vi "BuildCustomDashBoardData.vi"() -> ()   [LabVIEW 2013]
doc: "This VI builds data and sends it back to the dashboard PC program. By default it sends back the raw values for the first analog, digital, and solenoid module. Modify it to send back the data you want to view. Consider adding higher level data to the Dashboard Datatype.ctl and to this VI. Then update the Dashboard to display the data however you like.\n\nThis software is licensed. Open the labview\\readme\\WPI Robotics Library Open Source License.txt file for more information."
uses:
  typedefs/dashboard/DashboardEnable.ctl
  typedefs/test/test controls.ctl
  typedefs/fg_getset.ctl
  <vilib>/Rock Robotics/SystemInterfaces/Typedef/FPGA_TypedefDigitalModule.ctl
  <vilib>/Rock Robotics/WPI/DriverStation/WPI_DriverStationDigitalData.ctl
  typedefs/dashboard/misc dash data.ctl
  <vilib>/Rock Robotics/SystemInterfaces/System/FPGA_SystemGet.vi
  <vilib>/Rock Robotics/WPI/Compressor/WPI_CompressorGetSetRefNum.vi
  <vilib>/NI_Real-Time Target Support.lvlib
  typedefs/state machine/subStates.ctl
  typedefs/dashboard/custom dash data.ctl
  typedefs/dashboard/Dashboard Datatype.ctl
panel:
  out "Errors":errorcluster
  # "Generate Dashboard Data and Send it"
  # "Note: Test code calls some dashboard data, which is gotten there not here"
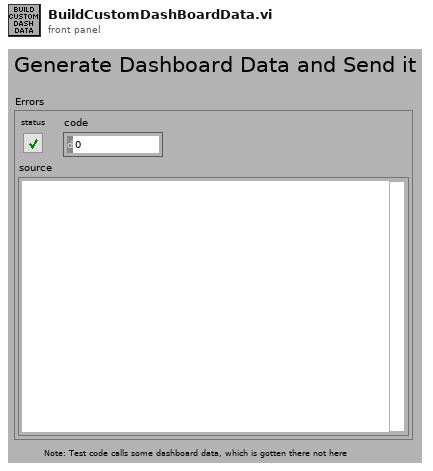
[diagram p1: front panel]
types:
  T1 = typedef "Dashboard Datatype.ctl" = cluster{cluster{"AnalogModule[0]":cluster{"Channel[0]":sgl, "Channel[1]":sgl, "Channel[2]":sgl, "Channel[3]":sgl, "Channel[4]":sgl, "Channel[5]":sgl, "Channel[6]":sgl, "Channel[7]":sgl}, "AnalogModule[1]":cluster{"Channel[0]":sgl, "Channel[1]":sgl, "Channel[2]":sgl, "Channel[3]":sgl, "Channel[4]":sgl, "Channel[5]":sgl, "Channel[6]":sgl, "Channel[7]":sgl}}, cluster{"DigitalModule[0]":T2, "DigitalModule[1]":T2}, "Solenoid":u8}
  T2 = typedef "WPI_DriverStationDigitalData.ctl" = cluster{"Relay Fwd":u8, "Relay Rev":u8, "GPIO":u16, "GPIO_OE":u16, "PWM":cluster{"PWM[0]":u8, "PWM[1]":u8, "PWM[2]":u8, "PWM[3]":u8, "PWM[4]":u8, "PWM[5]":u8, "PWM[6]":u8, "PWM[7]":u8, "PWM[8]":u8, "PWM[9]":u8}}
  T3 = typedef "custom dash data.ctl" = cluster{"Motors":cluster{"Pickup Motor":dbl, "Pickup Belt":dbl, "Pickup Distance ":dbl, "Pickup Rate":dbl, "Right Motor Rate":dbl, "Left Motor Rate":dbl, "Right Motor Distance":dbl, "Left Motor Distance":dbl}, "substates":cluster{"Latch":T4, "Pickup Arm":T4, "Belts":T4, "Shooter":T4, "Drive":T4}, "Safeties":cluster{"Arm Safety":bool, "Arm Limit":bool}, "Performance":cluster{"CPU Usage":dbl, "Vision mSPI":u32, "Main mSPI":u32}, "Vision Enabled?":bool, "Can Shoot Safely?":bool, "Timeout Error":cluster{"# of Timeouts":u32, "Time Out Error This Match":bool}, "Error FG Data":cluster{"Errors Present":bool, "Errors":string}, "Vision Data":cluster{"Hot Goal Present?":bool, "distance":dbl}}
  T4 = typedef "subStates.ctl" = enum16{"null", "wait", "driver control", "auto", "manual override", "hold position", "rotate", "test", "end"}
  T5 = typedef "fg_getset.ctl" = enum16{"Get", "Set"}
  T6 = cluster{"Hot Goal Present?":bool, "distance":dbl}
  T7 = typedef "test controls.ctl" = cluster{"Button":bool, "Switch":bool, "Slider":dbl}
  T8 = typedef "FPGA_TypedefDigitalModule.ctl" = enum16{"Digital Module 1", "Digital Module 2"}
  T9 = typedef "misc dash data.ctl" = cluster{"Total (%)":dbl, "Vision mSPI":u32, "Main mSPI":u32, "Vision":cluster{"distance":dbl}, "Enabled?":bool}
  T10 = typedef "DashboardEnable.ctl" = cluster{"Analog Module 1":bool[], "Analog Module 2":bool[], "Digital Module 1":bool, "Digital Module 2":bool, "Solenoid Module":bool}
  T11 = cluster{"AnalogModule[0]":cluster{"Channel[0]":sgl, "Channel[1]":sgl, "Channel[2]":sgl, "Channel[3]":sgl, "Channel[4]":sgl, "Channel[5]":sgl, "Channel[6]":sgl, "Channel[7]":sgl}, "AnalogModule[1]":cluster{"Channel[0]":sgl, "Channel[1]":sgl, "Channel[2]":sgl, "Channel[3]":sgl, "Channel[4]":sgl, "Channel[5]":sgl, "Channel[6]":sgl, "Channel[7]":sgl}}
  T12 = cluster{"DigitalModule[0]":T2, "DigitalModule[1]":T2}
  T13 = typedef "vision data.ctl" = cluster{"x":dbl, "y":dbl, "area":dbl, "width":dbl, "height":dbl}
  T14 = cluster{"Channel[0]":sgl, "Channel[1]":sgl, "Channel[2]":sgl, "Channel[3]":sgl, "Channel[4]":sgl, "Channel[5]":sgl, "Channel[6]":sgl, "Channel[7]":sgl}[]
  T15 = cluster{"Channel[0]":sgl, "Channel[1]":sgl, "Channel[2]":sgl, "Channel[3]":sgl, "Channel[4]":sgl, "Channel[5]":sgl, "Channel[6]":sgl, "Channel[7]":sgl}
  T16 = cluster{"AnalogModule[0][0]":sgl, "AnalogModule[0][1]":sgl, "AnalogModule[0][2]":sgl, "AnalogModule[0][3]":sgl, "AnalogModule[0][4]":sgl, "AnalogModule[0][5]":sgl, "AnalogModule[0][6]":sgl, "AnalogModule[0][7]":sgl}
  T17 = cluster{"[0]":cluster{"Channel[0]":sgl, "Channel[1]":sgl, "Channel[2]":sgl, "Channel[3]":sgl, "Channel[4]":sgl, "Channel[5]":sgl, "Channel[6]":sgl, "Channel[7]":sgl}, "[1]":cluster{"Channel[0]":sgl, "Channel[1]":sgl, "Channel[2]":sgl, "Channel[3]":sgl, "Channel[4]":sgl, "Channel[5]":sgl, "Channel[6]":sgl, "Channel[7]":sgl}}
  T18 = typedef "FPGA_DIODevRef.ctl" = cluster{"DevStatus":errorcluster, "Module":T8}
  T19 = cluster{"[0]":u8, "[1]":u8, "[2]":u8, "[3]":u8, "[4]":u8, "[5]":u8, "[6]":u8, "[7]":u8, "[8]":u8, "[9]":u8}
  T20 = typedef "FPGA_SolenoidDevRef.ctl" = cluster{"DevStatus":errorcluster, "Module":T21}
  T21 = typedef "FPGA_TypedefSolenoidModule.ctl" = enum16{"Solenoid Module 1", "Solenoid Module 2"}
  T22 = cluster{"Pickup Motor":dbl, "Pickup Belt":dbl, "Pickup Distance ":dbl, "Pickup Rate":dbl, "Right Motor Rate":dbl, "Left Motor Rate":dbl, "Right Motor Distance":dbl, "Left Motor Distance":dbl}
  T23 = cluster{"CPU Usage":dbl, "Vision mSPI":u32, "Main mSPI":u32}
  T24 = typedef "WPI_EncoderDevRef.ctl" = cluster{"DevStatus":errorcluster, "EncoderIndex":T25, "CounterIndex":T26, "DistancePerCount":dbl, "Decoding Type":T27}
  T25 = typedef "FPGA_EncoderIdx.ctl" = enum8{"Enc 0", "Enc 1", "Enc 2", "Enc 3", "Invalid"}
  T26 = typedef "FPGA_CounterCtrSystemIndex.ctl" = enum8{"Ctr 0", "Ctr 1", "Ctr 2", "Ctr 3", "Ctr 4", "Ctr 5", "Ctr 6", "Ctr 7", "Invalid"}
  T27 = typedef "WPI_EncoderType.ctl" = enum16{"1x", "2x", "4x"}
  T28 = typedef "WPI_MotorControlDeviceRef.ctl" = cluster{"DeviceStatus":errorcluster, "Type":enum16{"PWM", "CAN"}, "PWM":cluster{"Digital Module":T8, "PWM Channel":T29, "DeadBand":T30}, "CAN":cluster{"Device Number":u8, "Control Mode":T31, "Semaphore":T32, "Max Vout":dbl}, "Invert":bool, "TransformRef":T33, "InvTransformRef":T33}
  T29 = typedef "FPGA_DIOPWMChannel.ctl" = enum8{"PWM 1", "PWM 2", "PWM 3", "PWM 4", "PWM 5", "PWM 6", "PWM 7", "PWM 8", "PWM 9", "PWM 10", "Invalid"}
  T30 = typedef "WPI_PWMDeadband.ctl" = cluster{"Name":string, "maxPositivePwm":i32, "minPositivePwm":i32, "centerPwm":i32, "maxNegativePwm":i32, "minNegativePwm":i32, "angularRange":u16}
  T31 = typedef "WPI_CANJaguar_ControlMode.ctl" = enum8{"Percent VBus", "Current", "Speed", "Position", "Voltage"}
  T32 = typedef "Semaphore RefNum" = refnum<k1>
  T33 = typedef "WPI_PWMTransform_ConPane.ctl" = refnum<vi>
  T34 = typedef "NI_Real-Time Target Support.lvlib/RT CPU Load.ctl" = cluster{"Total (%)":dbl, "Time Critical (%)":dbl, "Timed Structures (%)":dbl, "High (%)":dbl, "Above Normal (%)":dbl, "Normal (%)":dbl, "Background (%)":dbl, "Idle (%)":dbl, "ISR (%)":dbl}
  T35 = cluster{"Vision mSPI":u32, "Main mSPI":u32, "Dash mSPI":u32}
  T36 = cluster{"# of Timeouts":u32, "Time Out Error This Match":bool}
  T37 = typedef "WPI_CompressorDevRef.ctl" = cluster{"DevStatus":errorcluster, "DigitalInputDevRef":T38, "RelayDevRef":T40}
  T38 = typedef "WPI_DigitalInputDevRef.ctl" = cluster{"DevStatus":errorcluster, "DIO Channel":T39, "Digital Module":T8}
  T39 = typedef "FPGA_DIOChannel.ctl" = enum8{"DIO 1", "DIO 2", "DIO 3", "DIO 4", "DIO 5", "DIO 6", "DIO 7", "DIO 8", "DIO 9", "DIO 10", "DIO 11", "DIO 12", "DIO 13", "DIO 14", "Invalid"}
  T40 = typedef "WPI_RelayDevRef.ctl" = cluster{"DevStatus":errorcluster, "Relay Channel":T41, "Digital Module":T8, "Relay Direction":T42}
  T41 = typedef "FPGA_DIORelayChannel.ctl" = enum8{"Relay 1", "Relay 2", "Relay 3", "Relay 4", "Relay 5", "Relay 6", "Relay 7", "Relay 8", "Invalid"}
  T42 = typedef "WPI_RelayDirection.ctl" = enum16{"Both directions", "Forward only", "Reverse only"}
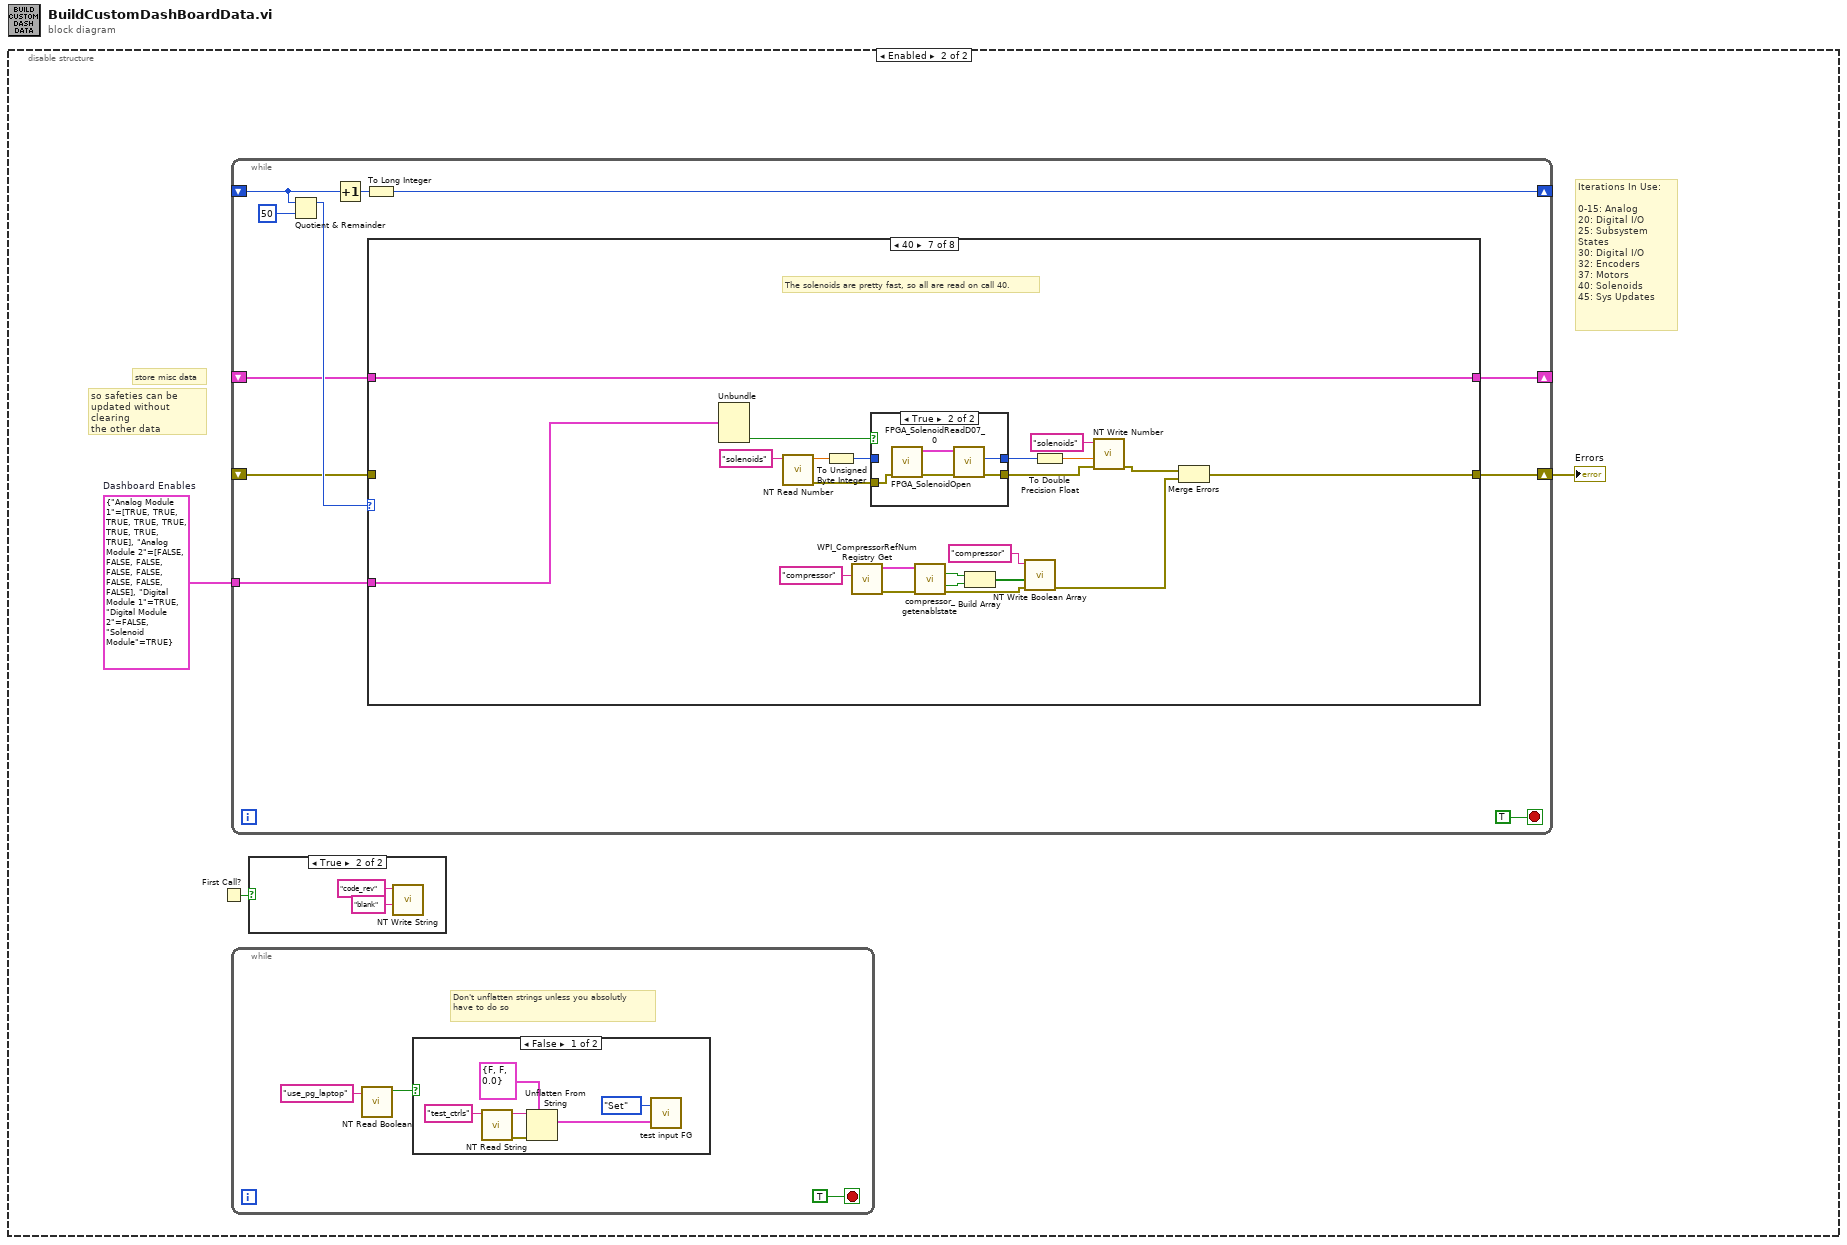
[diagram p0: block diagram]
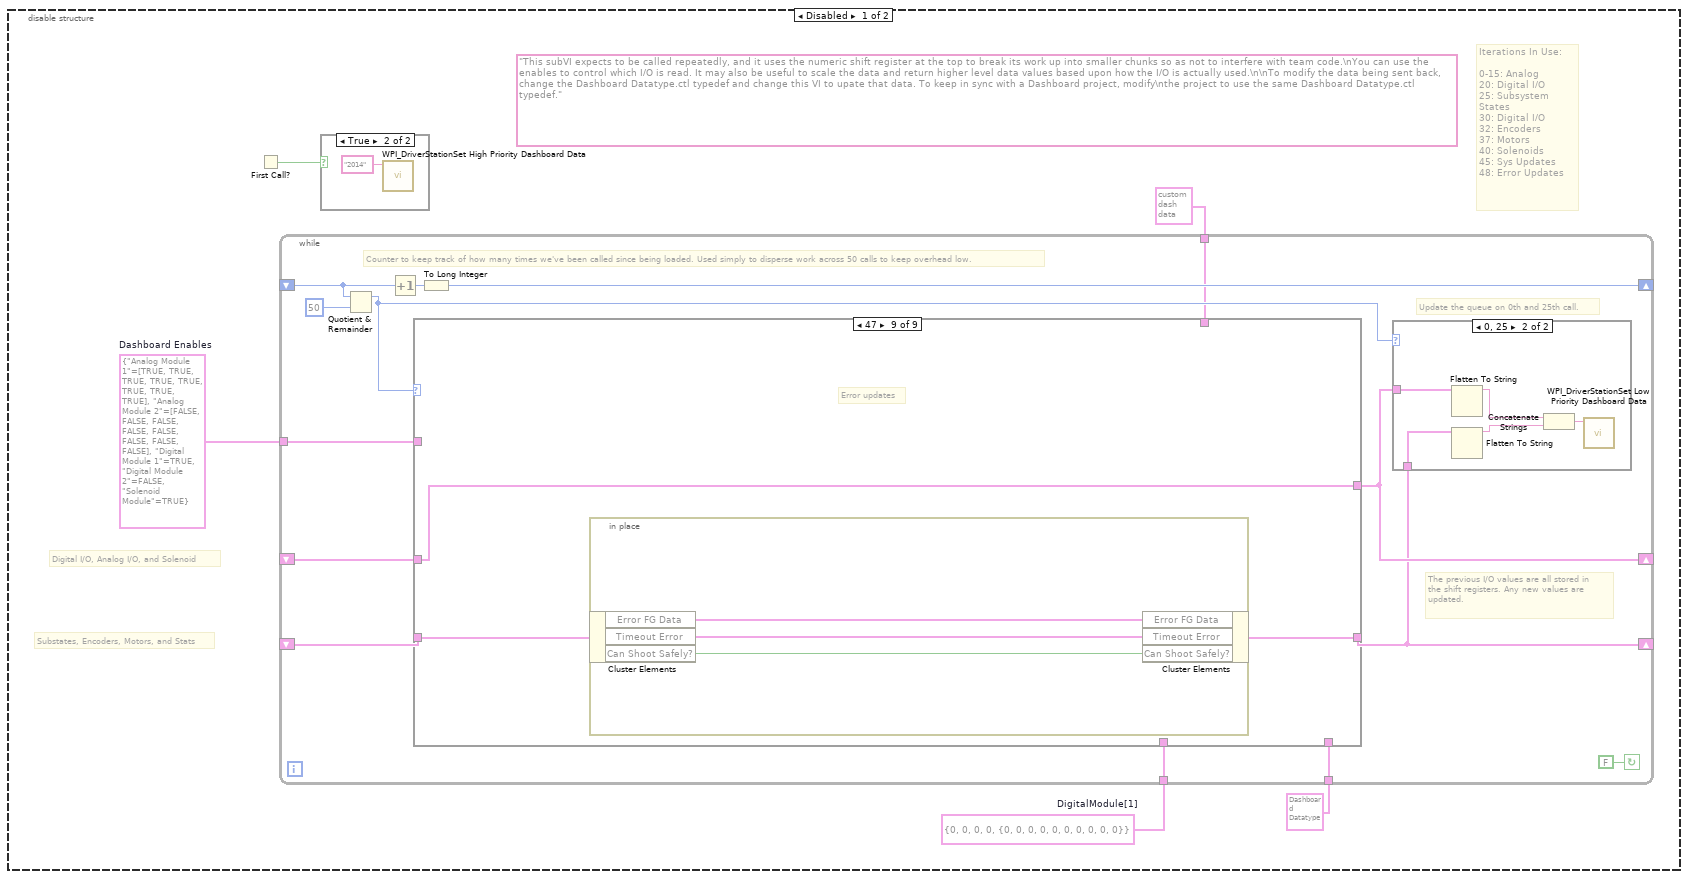
[diagram p2: hidden frame]
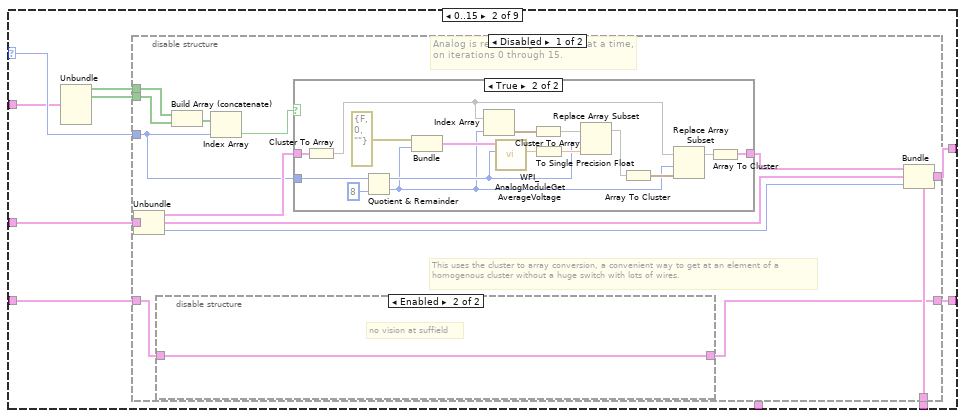
[diagram p6: hidden frame]
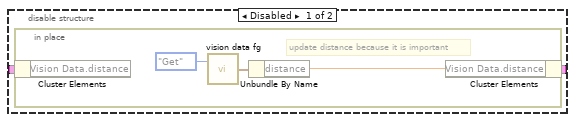
[diagram p8: hidden frame]
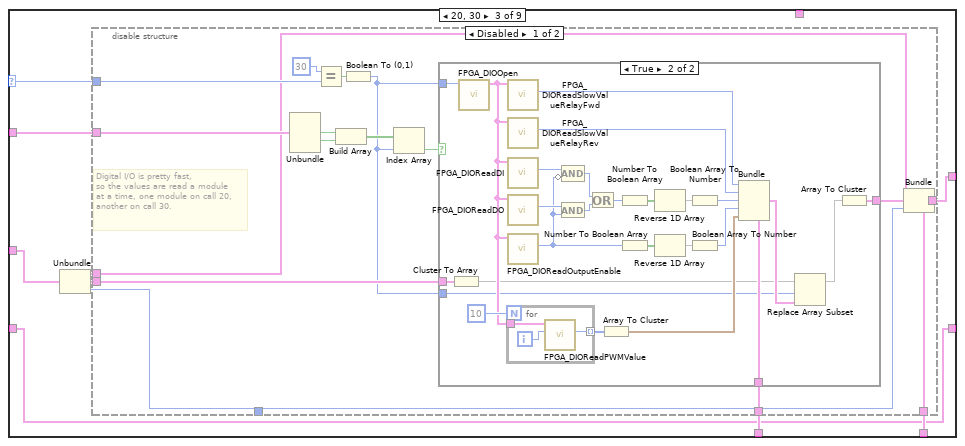
[diagram p10: hidden frame]
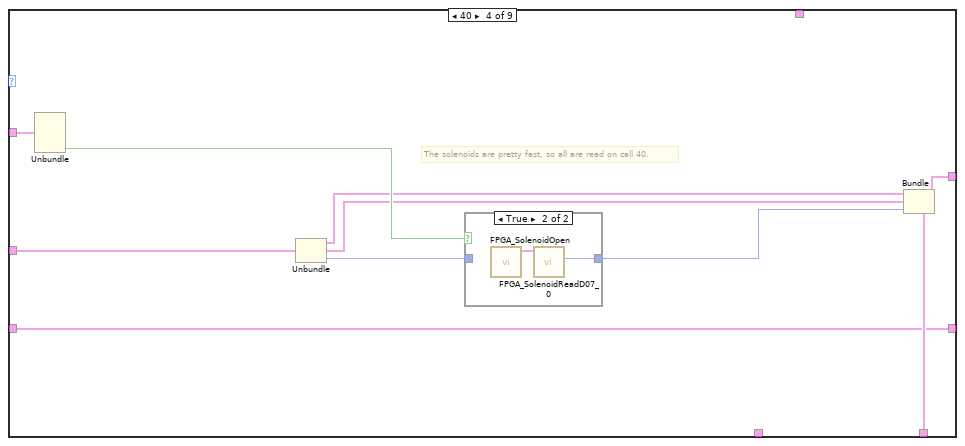
[diagram p13: hidden frame]
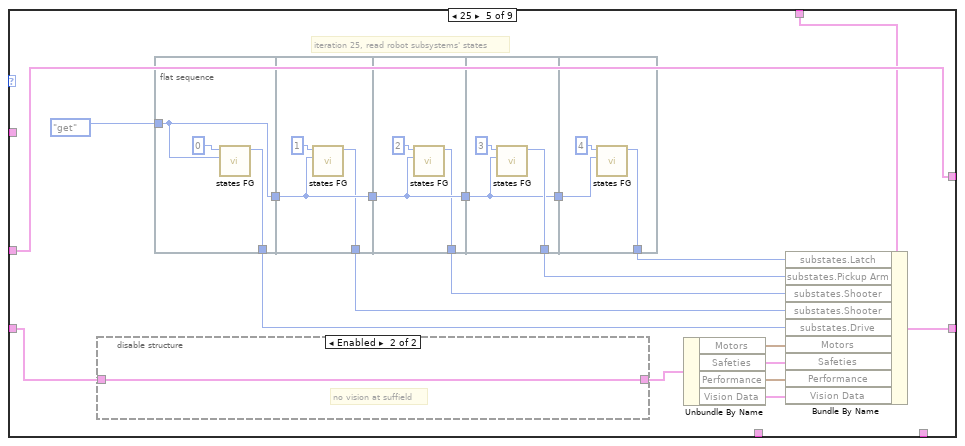
[diagram p15: hidden frame]
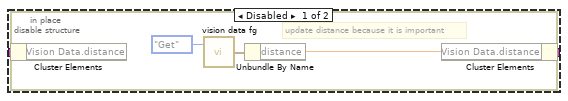
[diagram p16: hidden frame]
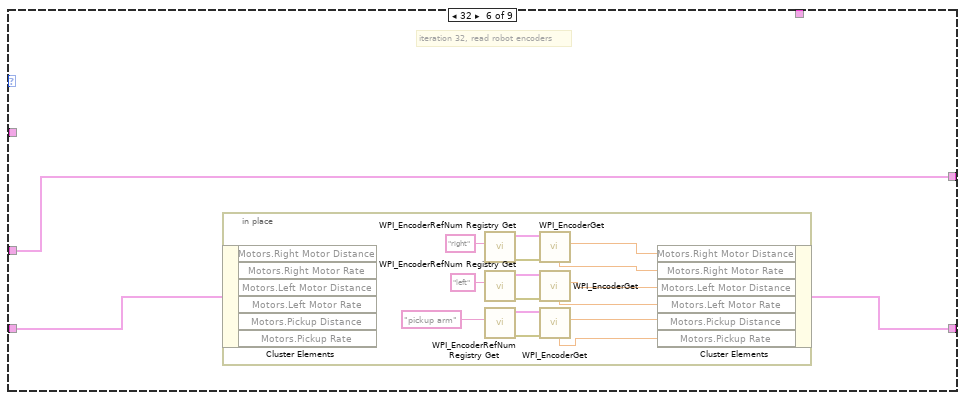
[diagram p17: hidden frame]
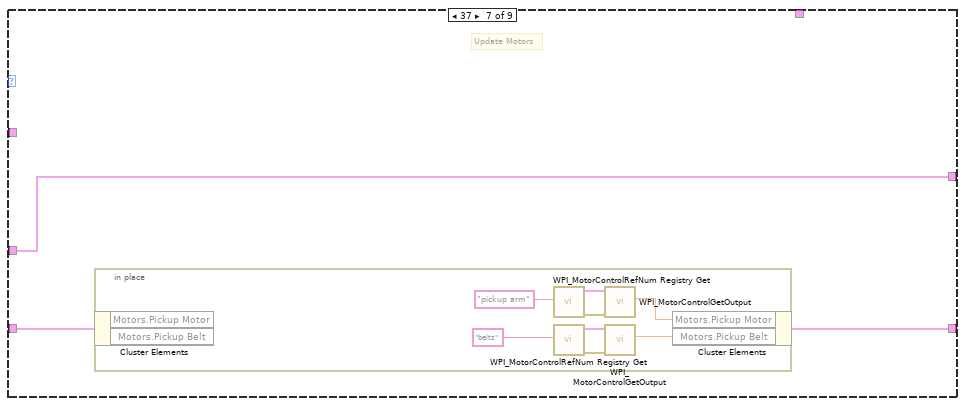
[diagram p18: hidden frame]
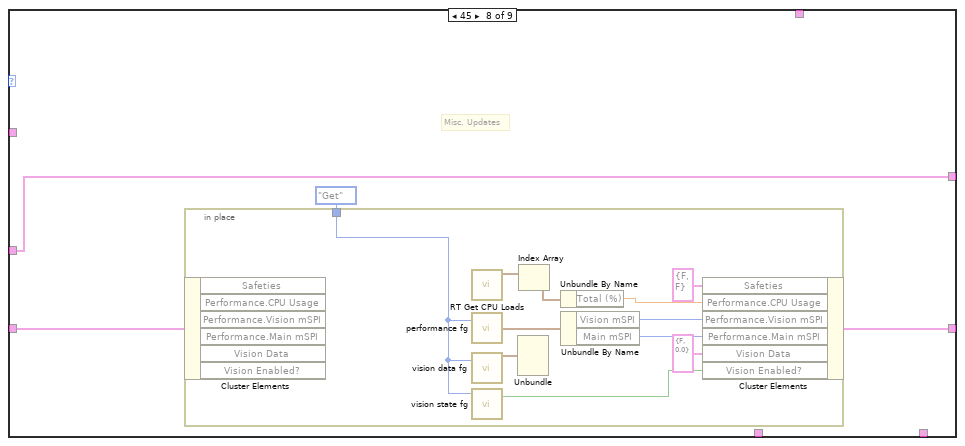
[diagram p19: hidden frame]
diagram:
  n1 = disable-structure shown="Enabled" {
    frame Disabled {
      w1 = T10 {"Analog Module 1"=[TRUE, TRUE, TRUE, TRUE, TRUE, TRUE, TRUE, TRUE], "Analog Module 2"=[FALSE, FALSE, FALSE, FALSE, FALSE, FALSE, FALSE, FALSE], "Digital Module 1"=TRUE, "Digital Module 2"=FALSE, "Solenoid Module"=TRUE}  # Dashboard Enables
      w2 = T2 {"Relay Fwd"=0, "Relay Rev"=0, "GPIO"=0, "GPIO_OE"=0, "PWM"={"PWM[0]"=0, "PWM[1]"=0, "PWM[2]"=0, "PWM[3]"=0, "PWM[4]"=0, "PWM[5]"=0, "PWM[6]"=0, "PWM[7]"=0, "PWM[8]"=0, "PWM[9]"=0}}  # DigitalModule[1]
      (unwired) "This subVI expects to be called repeatedly, and it uses the numeric shift register at the top to break its work up into smaller chunks so as not to interfere with team code.\nYou can use the enables to control which I/O is read. It may also be useful to scale the data and return higher level data values based upon how the I/O is actually used.\n\nTo modify the data being sent back, change the Dashboard Datatype.ctl typedef and change this VI to upate that data. To keep in sync with a Dashboard project, modify\nthe project to use the same Dashboard Datatype.ctl typedef."
      # "Iterations In Use:\n\n0-15: Analog\n20: Digital I/O \n25: Subsystem States\n30: Digital I/O\n32: Encoders\n37: Motors\n40: Solenoids\n45: Sys Updates\n48: Error Updates"
      # "Substates, Encoders, Motors, and Stats"
      # "Digital I/O, Analog I/O, and Solenoid"
      n2 = First Call?() -> (First Call?: T/F=w3:bool)
      n3 = while {
        shift-right: [w13] -> _
        shift-left: _ -> [w15]
        shift-right: [w10] -> _
        shift-left: _ -> [w18]
        tunnel: w2 -> [w17]
        tunnel: T1 {{"AnalogModule[0]"={"Channel[0]"=0.0, "Channel[1]"=0.0, "Channel[2]"=0.0, "Channel[3]"=0.0, "Channel[4]"=0.0, "Channel[5]"=0.0, "Channel[6]"=0.0, "Channel[7]"=0.0}, "AnalogModule[1]"={"Channel[0]"=0.0, "Channel[1]"=0.0, "Channel[2]"=0.0, "Channel[3]"=0.0, "Channel[4]"=0.0, "Channel[5]"=0.0, "Channel[6]"=0.0, "Channel[7]"=0.0}}, {"DigitalModule[0]"={"Relay Fwd"=0, "Relay Rev"=0, "GPIO"=0, "GPIO_OE"=0, "PWM"={"PWM[0]"=0, "PWM[1]"=0, "PWM[2]"=0, "PWM[3]"=0, "PWM[4]"=0, "PWM[5]"=0, "PWM[6]"=0, "PWM[7]"=0, "PWM[8]"=0, "PWM[9]"=0}}, "DigitalModule[1]"={"Relay Fwd"=0, "Relay Rev"=0, "GPIO"=0, "GPIO_OE"=0, "PWM"={"PWM[0]"=0, "PWM[1]"=0, "PWM[2]"=0, "PWM[3]"=0, "PWM[4]"=0, "PWM[5]"=0, "PWM[6]"=0, "PWM[7]"=0, "PWM[8]"=0, "PWM[9]"=0}}}, "Solenoid"=0} ("Dashboard Data") -> [w12]
        tunnel: w1 -> [w11]
        shift-right: [w7] -> _
        shift-left: _ -> [w8]
        tunnel: T3 {"Motors"={"Pickup Motor"=0.0, "Pickup Belt"=0.0, "Pickup Distance "=0.0, "Pickup Rate"=0.0, "Right Motor Rate"=0.0, "Left Motor Rate"=0.0, "Right Motor Distance"=0.0, "Left Motor Distance"=0.0}, "substates"={"Latch"=enum."null", "Pickup Arm"=enum."null", "Belts"=enum."null", "Shooter"=enum."null", "Drive"=enum."null"}, "Safeties"={"Arm Safety"=FALSE, "Arm Limit"=FALSE}, "Performance"={"CPU Usage"=0.0, "Vision mSPI"=0, "Main mSPI"=0}, "Vision Enabled?"=FALSE, "Can Shoot Safely?"=FALSE, "Timeout Error"={"# of Timeouts"=0, "Time Out Error This Match"=FALSE}, "Error FG Data"={"Errors Present"=FALSE, "Errors"=""}, "Vision Data"={"Hot Goal Present?"=FALSE, "distance"=0.0}} ("Custom Dash Data") -> [w9]
        stop <- FALSE continue-if-true
        # "Counter to keep track of how many times we've been called since being loaded. Used simply to disperse work across 50 calls to keep overhead low."
        # "Update the queue on 0th and 25th call."
        # "The previous I/O values are all stored in\nthe shift registers. Any new values are\nupdated."
        n4 = Quotient & Remainder(x=w15, y=50) -> (x-y*floor(x/y)=w14:i32)  [unwired: 1 out]
        n5 = Increment(x=w15) -> (x+1=w20:i32)
        n6 = case shown="47" w14 {
          selector: w14 -> [_ w35 w82 _ _ _ _ _ _]
          tunnel: [w27 w31 w77 w136 w151 w184 w203 w214 w228] -> w10
          tunnel: w18 -> [w27 w30 w79 w138 w151 w184 w203 w214 w228]
          tunnel: w17 -> [_ _ w83 _ _ _ _ _ _]
          tunnel: w12 -> [_ w36 w78 w135 _ _ _ _ _]
          tunnel: w11 -> [_ w34 w81 w139 _ _ _ _ _]
          tunnel: w9 -> [_ _ _ _ w149 _ _ _ _]
          tunnel: [w26 w28 w76 w132 w150 w185 w202 w215 w229] -> w7
          tunnel: w8 -> [w26 w29 w76 w132 w145 w183 w201 w213 w227]
          frame Default {
            # "Don't update any I/O"
          }
          frame 0..15 {
            n7 = Unbundle(w34) -> ("Analog Module 1"=w33:bool[], "Analog Module 2"=w32:bool[])  [unwired: 3 out]
            n8 = disable-structure shown="Disabled" {
              disable-tunnel: w36 -> [w47 _]
              disable-tunnel: w35 -> [w45 _]
              disable-tunnel: w33 -> [w44 _]
              disable-tunnel: w32 -> [w43 _]
              disable-tunnel: [w42 _] -> w31
              disable-tunnel: w30 -> [w41 _]
              disable-tunnel: w29 -> [w38 _]
              disable-tunnel: [w37 _] -> w28
              frame Disabled {
                # "This uses the cluster to array conversion, a convenient way to get at an element of a\nhomogenous cluster without a huge switch with lots of wires."
                # "Analog is read a single channel at a time,\non iterations 0 through 15."
                n9 = Unbundle(w41) -> (w46:T11, w40:T12, "Solenoid"=w39:u8)
                n10 = disable-structure shown="Enabled" {
                  disable-tunnel: w38 -> [w69 w73]
                  disable-tunnel: [w68 w73] -> w37
                  frame Disabled {
                    n11 = in-place {
                      # "update distance because it is important"
                      n12 = in-place-cluster #1(w69) -> ()  [unwired: 1 out]
                      n13 = call "vision data fg.vi"("Menu"=fg_getset."Get") -> ("Output"=w71:T13)  [unwired: 1 in]
                      n14 = Unbundle By Name(w71) -> ("distance"=w70:dbl)
                      n15 = in-place-cluster #1("Vision Data.distance"=w70) -> (w68:T3)
                    }
                  }
                  frame Enabled {
                    # "no vision at suffield"
                  }
                }
                n16 = Build Array (concatenate)(w44, w43) -> (w49:bool[])
                n17 = Index Array(array=w49, index=w45) -> (element=w50:bool)
                n18 = case shown="True" w50 {
                  tunnel: w45 -> [_ w58]
                  tunnel: [w51 w55] -> w48
                  tunnel: w46 -> [w51 w54]
                  frame False {
                  }
                  frame True {
                    n19 = Cluster To Array(cluster=w54) -> (array=w53:T14)
                    n20 = Quotient & Remainder(x=w58, y=8) -> (x-y*floor(x/y)=w57:i32, floor(x/y)=w52:i32)
                    n21 = Bundle("DevStatus"=errorcluster {"status"=FALSE, "code"=0, "source"=""}, w52) -> (w66:cluster{"DevStatus":errorcluster, i32})  [unwired: 1 out]
                    n22 = Index Array(array=w53, index=w52) -> (element=w60:T15)
                    n23 = call <vilib>:"WPI_AnalogModuleGetAverageVoltage.vi"("Channel"=w57, "AnalogModuleDevStatus"=w66) -> ("Average Voltage"=w63:dbl)  [unwired: 1 in, 8 out]
                    n24 = Cluster To Array(cluster=w60) -> (array=w59:sgl[])
                    n25 = To Single Precision Float(number=w63) -> (single precision float=w62:sgl)
                    n26 = Replace Array Subset(array=w59, new element=w62, index=w57) -> (w61:sgl[])
                    n27 = Array To Cluster(array=w61) -> (cluster=w65:T16)
                    n28 = Replace Array Subset(array=w53, new element=w65, index=w52) -> (w56:T14)
                    n29 = Array To Cluster(array=w56) -> (cluster=w55:T17)
                  }
                }
                n30 = Bundle(cluster=w47, w48, w40, "Solenoid"=w39) -> (w42:T1)
              }
              frame Enabled {
              }
            }
          }
          frame 20, 30 {
            n31 = Unbundle(w79) -> (w75:T11, w80:T12, "Solenoid"=w74:u8)
            n32 = disable-structure shown="Disabled" {
              disable-tunnel: w83 -> [w99 _]
              disable-tunnel: w82 -> [w95 _]
              disable-tunnel: w81 -> [w93 _]
              disable-tunnel: w80 -> [w90 _]
              disable-tunnel: w78 -> [w88 _]
              disable-tunnel: [w87 _] -> w77
              disable-tunnel: w75 -> [w85 _]
              disable-tunnel: w74 -> [w84 _]
              frame Disabled {
                # "Digital I/O is pretty fast,\nso the values are read a module\nat a time, one module on call 20,\nanother on call 30."
                n33 = Unbundle(w93) -> ("Digital Module 1"=w92:bool, "Digital Module 2"=w91:bool)  [unwired: 3 out]
                n34 = Equal?(x=30, y=w95) -> (x = y?=w97:bool)
                n35 = Build Array(w92, w91) -> (w94:bool[])
                n36 = Boolean To (0,1)(Boolean=w97) -> (0, 1=w86:i16)
                n37 = Index Array(array=w94, index=w86) -> (element=w96:bool)
                n38 = case shown="True" w96 {
                  tunnel: w99 -> [_ w108]
                  tunnel: [w100 w101] -> w89
                  tunnel: w86 -> [_ w106]
                  tunnel: w86 -> [_ w105]
                  tunnel: w90 -> [w100 w104]
                  frame False {
                  }
                  frame True {
                    n39 = Cluster To Array(cluster=w104) -> (array=w103:T2[])
                    n40 = call <vilib>:"FPGA_DIOOpen.vi"("Module (Module 1)"=w106) -> ("DIODeviceRef"=w124:T18)  [unwired: 1 in, 9 out]
                    n41 = for {
                      N: 10 -> [_]
                      tunnel: w124 -> [w129]
                      tunnel: [w127] -> w125 mode=indexing
                      i -> [w128]
                      n42 = call <vilib>:"FPGA_DIOReadPWMValue.vi"("PWMChannel"=w128, "DIODeviceRef In"=w129) -> ("PWMValue"=w127:u8)  [unwired: 1 in, 8 out]
                    }
                    n43 = call <vilib>:"FPGA_DIOReadSlowValueRelayFwd.vi"("DIODeviceRef In"=w124) -> ("Relay Forward"=w117:u8)  [unwired: 1 in, 9 out]
                    n44 = call <vilib>:"FPGA_DIOReadSlowValueRelayRev.vi"("DIODeviceRef In"=w124) -> ("Relay Reverse"=w118:u8)  [unwired: 1 in, 9 out]
                    n45 = call <vilib>:"FPGA_DIOReadDI.vi"("DIODeviceRef In"=w124) -> ("DI"=w122:u16)  [unwired: 1 in, 9 out]
                    n46 = call <vilib>:"FPGA_DIOReadDO.vi"("DIODeviceRef In"=w124) -> ("DO"=w121:u16)  [unwired: 1 in, 9 out]
                    n47 = call <vilib>:"FPGA_DIOReadOutputEnable.vi"("DIODeviceRef In"=w124) -> ("OutputEnable"=w112:u16)  [unwired: 1 in, 9 out]
                    n48 = And(x=w121, y=w112) -> (x .and. y?=w120:u16)
                    n49 = Compound Arithmetic op=AND(w122, invert w112) -> (w119:u16)
                    n50 = Or(x=w119, y=w120) -> (x .or. y?=w110:u16)
                    n51 = Array To Cluster(array=w125) -> (cluster=w123:T19)
                    n52 = Number To Boolean Array(number=w110) -> (Boolean array=w115:bool[])
                    n53 = Number To Boolean Array(number=w112) -> (Boolean array=w114:bool[])
                    n54 = Reverse 1D Array(array=w115) -> (reversed array=w116:bool[])
                    n55 = Reverse 1D Array(array=w114) -> (reversed array=w113:bool[])
                    n56 = Boolean Array To Number(Boolean array=w116) -> (number=w109:u32)
                    n57 = Boolean Array To Number(Boolean array=w113) -> (number=w111:u32)
                    n58 = Bundle(cluster=w108, "Relay Fwd"=w117, "Relay Rev"=w118, "GPIO"=w109, "GPIO_OE"=w111, "PWM"=w123) -> (w107:T2)
                    n59 = Replace Array Subset(array=w103, new element=w107, index=w105) -> (w102:T2[])
                    n60 = Array To Cluster(array=w102) -> (cluster=w101:cluster{"[0]":T2, "[1]":T2})
                  }
                }
                n61 = Bundle(cluster=w88, w85, w89, "Solenoid"=w84) -> (w87:T1)
              }
              frame Enabled {
              }
            }
          }
          frame 40 {
            # "The solenoids are pretty fast, so all are read on call 40."
            n62 = Unbundle(w139) -> ("Solenoid Module"=w133:bool)  [unwired: 4 out]
            n63 = Unbundle(w138) -> (w131:T11, w130:T12, "Solenoid"=w137:u8)
            n64 = case shown="True" w133 {
              tunnel: [w140 w141] -> w134
              tunnel: w137 -> [w140 _]
              frame False {
              }
              frame True {
                n65 = call <vilib>:"FPGA_SolenoidOpen.vi"() -> ("SolenoidDevRef"=w142:T20)  [unwired: 2 in, 9 out]
                n66 = call <vilib>:"FPGA_SolenoidReadD07_0.vi"("SolenoidDevRef"=w142) -> ("DO7:0"=w141:u8)  [unwired: 1 in, 9 out]
              }
            }
            n67 = Bundle(cluster=w135, w131, w130, "Solenoid"=w134) -> (w136:T1)
          }
          frame 25 {
            # "iteration 25, read robot subsystems' states"
            n68 = disable-structure shown="Enabled" {
              disable-tunnel: w145 -> [w163 w167]
              disable-tunnel: [w162 w167] -> w144
              frame Disabled {
                n69 = in-place {
                  # "update distance because it is important"
                  n70 = in-place-cluster #2(w163) -> ()  [unwired: 1 out]
                  n71 = call "vision data fg.vi"("Menu"=fg_getset."Get") -> ("Output"=w165:T13)  [unwired: 1 in]
                  n72 = Unbundle By Name(w165) -> ("distance"=w164:dbl)
                  n73 = in-place-cluster #2("Vision Data.distance"=w164) -> (w162:T3)
                }
              }
              frame Enabled {
                # "no vision at suffield"
              }
            }
            n74 = flat-sequence {
              tunnel: enum16{"set", "get"}."get" ("menu (get)") -> [w170]
              tunnel: [w170] -> w158
              tunnel: [w168] -> w152
              tunnel: [w173] -> w159
              tunnel: w158 -> [w173]
              tunnel: [w171] -> w153
              tunnel: [w176] -> w160
              tunnel: w159 -> [w176]
              tunnel: [w174] -> w154
              tunnel: w160 -> [w177]
              tunnel: [w178] -> w155
              tunnel: [w177] -> w157
              tunnel: w157 -> [w181]
              tunnel: [w180] -> w156
              frame #0 {
                n75 = call "states FG.vi"("menu (get)"=w170, "Loop ID"=0) -> ("subState out"=w168:T4)  [unwired: 6 in, 3 out]
              }
              frame #1 {
                n76 = call "states FG.vi"("menu (get)"=w173, "Loop ID"=1) -> ("subState out"=w171:T4)  [unwired: 6 in, 3 out]
              }
              frame #2 {
                n77 = call "states FG.vi"("menu (get)"=w176, "Loop ID"=2) -> ("subState out"=w174:T4)  [unwired: 6 in, 3 out]
              }
              frame #3 {
                n78 = call "states FG.vi"("menu (get)"=w177, "Loop ID"=3) -> ("subState out"=w178:T4)  [unwired: 6 in, 3 out]
              }
              frame #4 {
                n79 = call "states FG.vi"("menu (get)"=w181, "Loop ID"=4) -> ("subState out"=w180:T4)  [unwired: 6 in, 3 out]
              }
            }
            n80 = Unbundle By Name(w144) -> ("Motors"=w143:T22, "Safeties"=w148:cluster{"Arm Safety":bool, "Arm Limit":bool}, "Performance"=w147:T23, "Vision Data"=w146:T6)
            n81 = Bundle By Name(cluster=w149, "substates.Latch"=w156, "substates.Pickup Arm"=w155, "substates.Shooter"=w154, "substates.Shooter"=w153, "substates.Drive"=w152, "Motors"=w143, "Safeties"=w148, "Performance"=w147, "Vision Data"=w146) -> (w150:T3)
          }
          frame 32 {
            # "iteration 32, read robot encoders"
            n82 = in-place {
              n83 = in-place-cluster #3(w183) -> ()  [unwired: 6 out]
              n84 = call <vilib>:"WPI_EncoderRefNum Registry Get.vi"("refnum name"="right") -> ("error out"=w192:errorcluster, "EncoderDevRef"=w193:T24)  [unwired: 9 in]
              n85 = call <vilib>:"WPI_EncoderRefNum Registry Get.vi"("refnum name"="left") -> ("error out"=w195:errorcluster, "EncoderDevRef"=w194:T24)  [unwired: 9 in]
              n86 = call <vilib>:"WPI_EncoderRefNum Registry Get.vi"("refnum name"="pickup arm") -> ("error out"=w199:errorcluster, "EncoderDevRef"=w200:T24)  [unwired: 9 in]
              n87 = call <vilib>:"WPI_EncoderGet.vi"("error in (no error)"=w192, "EncoderDevRef"=w193) -> ("Distance"=w187:dbl, "Rate"=w186:dbl)  [unwired: 4 in, 4 out]
              n88 = call <vilib>:"WPI_EncoderGet.vi"("error in (no error)"=w195, "EncoderDevRef"=w194) -> ("Distance"=w188:dbl, "Rate"=w189:dbl)  [unwired: 4 in, 4 out]
              n89 = call <vilib>:"WPI_EncoderGet.vi"("error in (no error)"=w199, "EncoderDevRef"=w200) -> ("Distance"=w197:dbl, "Rate"=w196:dbl)  [unwired: 4 in, 4 out]
              n90 = in-place-cluster #3("Motors.Right Motor Distance"=w187, "Motors.Right Motor Rate"=w186, "Motors.Left Motor Distance"=w188, "Motors.Left Motor Rate"=w189, "Motors.Pickup Distance"=w197, "Motors.Pickup Rate"=w196) -> (w185:T3)
            }
          }
          frame 37 {
            # "Update Motors"
            n91 = in-place {
              n92 = in-place-cluster #4(w201) -> ()  [unwired: 2 out]
              n93 = call <vilib>:"WPI_MotorControlRefNum Registry Get.vi"("refnum name"="pickup arm") -> ("error out"=w204:errorcluster, "MotorControlDevRef"=w208:T28)  [unwired: 9 in]
              n94 = call <vilib>:"WPI_MotorControlRefNum Registry Get.vi"("refnum name"="belts") -> ("error out"=w205:errorcluster, "MotorControlDevRef"=w211:T28)  [unwired: 9 in]
              n95 = call <vilib>:"WPI_MotorControlGetOutput.vi"("error in (no error)"=w204, "MotorControlDevRef"=w208) -> ("Output"=w207:dbl)  [unwired: 7 in, 2 out]
              n96 = call <vilib>:"WPI_MotorControlGetOutput.vi"("error in (no error)"=w205, "MotorControlDevRef"=w211) -> ("Output"=w206:dbl)  [unwired: 7 in, 2 out]
              n97 = in-place-cluster #4("Motors.Pickup Motor"=w207, "Motors.Pickup Belt"=w206) -> (w202:T3)
            }
          }
          frame 45 {
            # "Misc. Updates"
            n98 = in-place {
              in-place-border: fg_getset."Get" ("Menu (Get)") -> [w219]
              n99 = in-place-cluster #5(w213) -> ()  [unwired: 6 out]
              n100 = call <vilib>:"RT Get CPU Loads.vi"() -> ("CPU loads"=w225:T34[])  [unwired: 10 in, 1 out]
              n101 = call "performance fg.vi"("Menu"=w219) -> ("Output"=w221:T35)  [unwired: 1 in]
              n102 = call "vision data fg.vi"("Menu"=w219) -> ("Output"=w218:T13)  [unwired: 1 in]
              n103 = call "vision state fg.vi"("Menu"=w219) -> ("Enabled?"=w220:bool)  [unwired: 2 in, 1 out]
              n104 = Unbundle(w218) -> ()  [unwired: 5 out]
              n105 = Index Array(array=w225) -> (element=w226:T34)  [unwired: 1 in]
              n106 = Unbundle By Name(w226) -> ("Total (%)"=w224:dbl)
              n107 = Unbundle By Name(w221) -> ("Vision mSPI"=w223:u32, "Main mSPI"=w222:u32)
              n108 = in-place-cluster #5("Safeties"=cluster{"Arm Safety":bool, "Arm Limit":bool} {"Arm Safety"=FALSE, "Arm Limit"=FALSE}, "Performance.CPU Usage"=w224, "Performance.Vision mSPI"=w223, "Performance.Main mSPI"=w222, "Vision Data"=T6 {"Hot Goal Present?"=FALSE, "distance"=0.0}, "Vision Enabled?"=w220) -> (w215:T3)
            }
          }
          frame 47 {
            # "Error updates"
            n109 = in-place {
              n110 = in-place-cluster #6(w227) -> ("Error FG Data"=w230:cluster{"Errors Present":bool, "Errors":string}, "Timeout Error"=w231:T36, "Can Shoot Safely?"=w232:bool)
              n111 = in-place-cluster #6("Error FG Data"=w230, "Timeout Error"=w231, "Can Shoot Safely?"=w232) -> (w229:T3)
            }
          }
        }
        n112 = To Long Integer(number=w20) -> (32bit integer=w13:i32)
        n113 = case shown="0, 25" w14 {
          tunnel: w10 -> [_ w25]
          tunnel: w7 -> [_ w23]
          frame Default {
          }
          frame 0, 25 {
            n114 = Flatten To String(anything=w25) -> (data string=w24:string)  [unwired: 1 in, 4 out]
            n115 = Flatten To String(anything=w23) -> (data string=w21:string)  [unwired: 1 in, 4 out]
            n116 = Concatenate Strings(w24, w21) -> (w22:string)
            n117 = call <vilib>:"WPI_DriverStationSet Low Priority Dashboard Data.vi"("User Data"=w22) -> ()  [unwired: 1 in, 10 out]
          }
        }
      }
      n118 = case shown="True" w3 {
        frame False {
        }
        frame True {
          n119 = call <vilib>:"WPI_DriverStationSet High Priority Dashboard Data.vi"("User Data"="2014") -> ()  [unwired: 10 in, 1 out]
        }
      }
    }
    frame Enabled {
      w235 = T10 {"Analog Module 1"=[TRUE, TRUE, TRUE, TRUE, TRUE, TRUE, TRUE, TRUE], "Analog Module 2"=[FALSE, FALSE, FALSE, FALSE, FALSE, FALSE, FALSE, FALSE], "Digital Module 1"=TRUE, "Digital Module 2"=FALSE, "Solenoid Module"=TRUE}  # Dashboard Enables
      # "so safeties can be\nupdated without clearing\nthe other data"
      # "store misc data"
      # "Iterations In Use:\n\n0-15: Analog\n20: Digital I/O \n25: Subsystem States\n30: Digital I/O\n32: Encoders\n37: Motors\n40: Solenoids\n45: Sys Updates"
      n120 = First Call?() -> (First Call?: T/F=w233:bool)
      n121 = while {
        shift-right: [w254] -> _
        shift-left: _ -> [w255]
        tunnel: w235 -> [w252]
        shift-right: [w250] -> w234
        shift-left: _ -> [w249]
        shift-right: [w248] -> _
        shift-left: _ -> [w247]
        stop <- TRUE stop-if-true
        n122 = Quotient & Remainder(x=w255, y=50) -> (x-y*floor(x/y)=w251:i32)  [unwired: 1 out]
        n123 = Increment(x=w255) -> (x+1=w256:i32)
        n124 = To Long Integer(number=w256) -> (32bit integer=w254:i32)
        n125 = case shown="40" w251 {
          selector: w251 -> [_ w268 _ w323 _ _ _ _]
          tunnel: w252 -> [_ w269 _ w322 _ _ w407 _]
          tunnel: [w259 w267 w288 w313 w371 w385 w389 w416] -> w250
          tunnel: w249 -> [w259 w266 w287 w314 _ w385 _ _]
          tunnel: [w258 w260 w286 w312 w372 w386 w398 w418] -> w248
          tunnel: w247 -> [w258 w260 w286 w312 w372 w386 w398 _]
          frame Default {
          }
          frame 0..15 {
            # "Analog is read a single channel at a time,\non iterations 0 through 15."
            n126 = Unbundle(w269) -> ("Analog Module 1"=w264:bool[], "Analog Module 2"=w265:bool[])  [unwired: 3 out]
            n127 = Build Array (concatenate)(w264, w265) -> (w262:bool[])
            n128 = Index Array(array=w262, index=w268) -> (element=w263:bool)
            n129 = case shown="True" w263 {
              tunnel: w268 -> [_ w281]
              tunnel: [w270 w271] -> w261
              tunnel: w266 -> [w270 _]
              frame False {
              }
              frame True {
                n130 = Quotient & Remainder(x=w281, y=8) -> (x-y*floor(x/y)=w278:i32, floor(x/y)=w282:i32)
                n131 = Bundle("DevStatus"=errorcluster {"status"=FALSE, "code"=0, "source"=""}, w282) -> (w284:cluster{"DevStatus":errorcluster, i32})  [unwired: 1 out]
                n132 = call <vilib>:"NT Read Numeric Array.vi"("Name"="analog") -> ("error out"=w273:errorcluster, "Numeric Array"=w279:dbl[])  [unwired: 9 in]
                n133 = call <vilib>:"WPI_AnalogModuleGetAverageVoltage.vi"("Channel"=w278, "AnalogModuleDevStatus"=w284) -> ("error out"=w272:errorcluster, "Average Voltage"=w277:dbl)  [unwired: 1 in, 7 out]
                n134 = Replace Array Subset(array=w279, new element=w277, index=w278) -> (w275:dbl[])
                n135 = Merge Errors(w273, w272) -> (w274:errorcluster)
                n136 = call <vilib>:"NT Write Numeric Array.vi"("error in"=w274, "Numeric Array"=w275, "Name"="analog") -> ("error out"=w271:errorcluster)  [unwired: 8 in]
              }
            }
            n137 = Merge Errors(w261, w266) -> (w267:errorcluster)
          }
          frame 25 {
            w302 = enum16{"set", "get"}."get" ("menu (get)")
            # "update subsystem states"
            n138 = call "states FG.vi"("menu (get)"=w302, "Loop ID"=0) -> ("subState out"=w299:T4)  [unwired: 6 in, 3 out]
            n139 = call "states FG.vi"("menu (get)"=w302, "Loop ID"=1) -> ("subState out"=w300:T4)  [unwired: 6 in, 3 out]
            n140 = call "states FG.vi"("menu (get)"=w302, "Loop ID"=2) -> ("subState out"=w301:T4)  [unwired: 6 in, 3 out]
            n141 = call "states FG.vi"("menu (get)"=w302, "Loop ID"=3) -> ("subState out"=w298:T4)  [unwired: 6 in, 3 out]
            n142 = call "states FG.vi"("menu (get)"=w302, "Loop ID"=4) -> ("subState out"=w297:T4)  [unwired: 6 in, 3 out]
            n143 = To Double Precision Float(number=w299) -> (double precision float=w295:dbl)
            n144 = To Double Precision Float(number=w300) -> (double precision float=w294:dbl)
            n145 = To Double Precision Float(number=w301) -> (double precision float=w293:dbl)
            n146 = To Double Precision Float(number=w298) -> (double precision float=w292:dbl)
            n147 = To Double Precision Float(number=w297) -> (double precision float=w291:dbl)
            n148 = Build Array(w295, w294, w293, w292, w291) -> (w290:dbl[])
            n149 = call <vilib>:"NT Write Numeric Array.vi"("Numeric Array"=w290, "Name"="subsystem_states") -> ("error out"=w289:errorcluster)  [unwired: 9 in]
            n150 = disable-structure shown="Enabled" {
              disable-tunnel: w289 -> [w310 _]
              disable-tunnel: [w309 w311] -> w288
              disable-tunnel: w287 -> [w308 w311]
              frame Disabled {
                n151 = Merge Errors(w310, w308) -> (w309:errorcluster)
              }
              frame Enabled {
              }
            }
          }
          frame 20, 30 {
            # "Digital I/O is pretty fast,\nso the values are read a module\nat a time, one module on call 20,\nanother on call 30."
            n152 = Equal?(x=30, y=w323) -> (x = y?=w320:bool)
            n153 = Boolean To (0,1)(Boolean=w320) -> (0, 1=w321:i16)
            n154 = Unbundle(w322) -> ("Digital Module 1"=w325:bool, "Digital Module 2"=w324:bool)  [unwired: 3 out]
            n155 = To Long Integer(number=w321) -> (32bit integer=w318:i32)
            n156 = Select(t=FPGA_TypedefDigitalModule."Digital Module 2" ("Module (Module 1)"), s=w320, f=FPGA_TypedefDigitalModule."Digital Module 1" ("Module (Module 1)")) -> (s? t:f=w317:T8)
            n157 = Build Array(w325, w324) -> (w326:bool[])
            n158 = Index Array(array=w326, index=w318) -> (element=w327:bool)
            n159 = case shown="True" w327 {
              tunnel: w317 -> [_ w343]
              tunnel: w318 -> [_ w342]
              tunnel: [errorcluster {"status"=FALSE, "code"=0, "source"=""} ("error out") w337] -> w315
              tunnel: w314 -> [_ _]
              frame False {
              }
              frame True {
                n160 = call <vilib>:"FPGA_DIOOpen.vi"("Module (Module 1)"=w343) -> ("DIODeviceRef"=w360:T18)  [unwired: 1 in, 9 out]
                n161 = for {
                  N: 10 -> [_]
                  tunnel: w360 -> [w370]
                  tunnel: [w368] -> w361 mode=indexing
                  i -> [w369]
                  n162 = To Unsigned Byte Integer(number=w369) -> (unsigned 8bit integer=w367:u8)
                  n163 = call <vilib>:"FPGA_DIOReadPWMValue.vi"("PWMChannel"=w367, "DIODeviceRef In"=w370) -> ("PWMValue"=w368:u8)  [unwired: 1 in, 8 out]
                }
                n164 = call <vilib>:"FPGA_DIOReadSlowValueRelayFwd.vi"("DIODeviceRef In"=w360) -> ("Relay Forward"=w353:u8)  [unwired: 1 in, 9 out]
                n165 = call <vilib>:"FPGA_DIOReadSlowValueRelayRev.vi"("DIODeviceRef In"=w360) -> ("Relay Reverse"=w354:u8)  [unwired: 1 in, 9 out]
                n166 = call <vilib>:"FPGA_DIOReadDI.vi"("DIODeviceRef In"=w360) -> ("DI"=w358:u16)  [unwired: 1 in, 9 out]
                n167 = call <vilib>:"FPGA_DIOReadDO.vi"("DIODeviceRef In"=w360) -> ("DO"=w357:u16)  [unwired: 1 in, 9 out]
                n168 = call <vilib>:"FPGA_DIOReadOutputEnable.vi"("DIODeviceRef In"=w360) -> ("OutputEnable"=w348:u16)  [unwired: 1 in, 9 out]
                n169 = And(x=w357, y=w348) -> (x .and. y?=w356:u16)
                n170 = Compound Arithmetic op=AND(w358, invert w348) -> (w355:u16)
                n171 = Number To Boolean Array(number=w348) -> (Boolean array=w350:bool[])
                n172 = Or(x=w355, y=w356) -> (x .or. y?=w346:u16)
                n173 = Reverse 1D Array(array=w350) -> (reversed array=w349:bool[])
                n174 = Number To Boolean Array(number=w346) -> (Boolean array=w351:bool[])
                n175 = Boolean Array To Number(Boolean array=w349) -> (number=w347:u32)
                n176 = Reverse 1D Array(array=w351) -> (reversed array=w352:bool[])
                n177 = Array To Cluster(array=w361) -> (cluster=w359:T19)
                n178 = Boolean Array To Number(Boolean array=w352) -> (number=w345:u32)
                n179 = To Unsigned Word Integer(number=w345) -> (unsigned 16bit integer=w334:u16)
                n180 = To Unsigned Word Integer(number=w347) -> (unsigned 16bit integer=w335:u16)
                n181 = Bundle(cluster=T2 {"Relay Fwd"=0, "Relay Rev"=0, "GPIO"=0, "GPIO_OE"=0, "PWM"={"PWM[0]"=0, "PWM[1]"=0, "PWM[2]"=0, "PWM[3]"=0, "PWM[4]"=0, "PWM[5]"=0, "PWM[6]"=0, "PWM[7]"=0, "PWM[8]"=0, "PWM[9]"=0}} ("DigitalModule"), "Relay Fwd"=w353, "Relay Rev"=w354, "GPIO"=w334, "GPIO_OE"=w335, "PWM"=w359) -> (w344:T2)
                n182 = disable-structure shown="Enabled" {
                  disable-tunnel: w344 -> [w365 w366]
                  disable-tunnel: w342 -> [w364 _]
                  disable-tunnel: [_ w366] -> w341
                  frame Disabled {
                    n183 = Replace Array Subset(array=T2[] [], new element=w365, index=w364) -> ()  [unwired: 1 out]
                  }
                  frame Enabled {
                  }
                }
                n184 = Flatten To String(anything=w341) -> (data string=w339:string, error out=w340:errorcluster)  [unwired: 1 in, 3 out]
                n185 = call <vilib>:"NT Write String.vi"("error in"=w340, "String"=w339, "Name"="dio") -> ("error out"=w337:errorcluster)  [unwired: 8 in]
              }
            }
            n186 = disable-structure shown="Enabled" {
              disable-tunnel: w315 -> [w331 _]
              disable-tunnel: w314 -> [w330 w332]
              disable-tunnel: [w329 w332] -> w313
              frame Disabled {
                n187 = Merge Errors(w331, w330) -> (w329:errorcluster)
              }
              frame Enabled {
              }
            }
          }
          frame 32 {
            # "update encoders"
            n188 = call <vilib>:"WPI_EncoderRefNum Registry Get.vi"("refnum name"="right") -> ("error out"=w382:errorcluster, "EncoderDevRef"=w381:T24)  [unwired: 9 in]
            n189 = call <vilib>:"WPI_EncoderRefNum Registry Get.vi"("refnum name"="left") -> ("error out"=w379:errorcluster, "EncoderDevRef"=w380:T24)  [unwired: 9 in]
            n190 = call <vilib>:"WPI_EncoderGet.vi"("error in (no error)"=w382, "EncoderDevRef"=w381) -> ("Distance"=w377:dbl, "Rate"=w376:dbl)  [unwired: 4 in, 4 out]
            n191 = call <vilib>:"WPI_EncoderGet.vi"("error in (no error)"=w379, "EncoderDevRef"=w380) -> ("Distance"=w375:dbl, "Rate"=w374:dbl)  [unwired: 4 in, 4 out]
            n192 = Build Array(w377, w376, w375, w374) -> (w373:dbl[])
            n193 = call <vilib>:"NT Write Numeric Array.vi"("Numeric Array"=w373, "Name"="encoders") -> ("error out"=w371:errorcluster)  [unwired: 9 in]
          }
          frame 37 {
            # "update motor array"
          }
          frame 40 {
            # "The solenoids are pretty fast, so all are read on call 40."
            n194 = Unbundle(w407) -> ("Solenoid Module"=w408:bool)  [unwired: 4 out]
            n195 = call <vilib>:"NT Read Number.vi"("Name"="solenoids") -> ("error out"=w399:errorcluster, "Numeric"=w404:dbl)  [unwired: 9 in]
            n196 = To Unsigned Byte Integer(number=w404) -> (unsigned 8bit integer=w402:u8)
            n197 = call <vilib>:"WPI_CompressorRefNum Registry Get.vi"("refnum name"="compressor") -> ("error out"=w397:errorcluster, "CompressorDevRef"=w396:T37)  [unwired: 9 in]
            n198 = case shown="True" w408 {
              tunnel: [w410 w414] -> w406
              tunnel: w402 -> [w410 _]
              tunnel: [w409 w412] -> w400
              tunnel: w399 -> [w409 w411]
              frame False {
              }
              frame True {
                n199 = call <vilib>:"FPGA_SolenoidOpen.vi"("error in (no error)"=w411) -> ("error out"=w413:errorcluster, "SolenoidDevRef"=w415:T20)  [unwired: 1 in, 8 out]
                n200 = call <vilib>:"FPGA_SolenoidReadD07_0.vi"("error in (no error)"=w413, "SolenoidDevRef"=w415) -> ("error out"=w412:errorcluster, "DO7:0"=w414:u8)  [unwired: 8 out]
              }
            }
            n201 = call "compressor_getenablstate.vi"("CompressorDevRef"=w396, "error in (no error)"=w397) -> ("Enabled"=w394:bool, "Compressor Running"=w393:bool, "error out"=w390:errorcluster)  [unwired: 7 in, 4 out]
            n202 = Build Array(w394, w393) -> (w392:bool[])
            n203 = call <vilib>:"NT Write Boolean Array.vi"("error in"=w390, "Boolean Array"=w392, "Name"="compressor") -> ("error out"=w388:errorcluster)  [unwired: 8 in]
            n204 = To Double Precision Float(number=w406) -> (double precision float=w401:dbl)
            n205 = call <vilib>:"NT Write Number.vi"("error in"=w400, "Numeric"=w401, "Name"="solenoids") -> ("error out"=w387:errorcluster)  [unwired: 8 in]
            n206 = Merge Errors(w387, w388) -> (w389:errorcluster)
          }
          frame 45 {
            w428 = fg_getset."Get" ("Menu")
            n207 = call <vilib>:"RT Get CPU Loads.vi"() -> ("error out"=w419:errorcluster, "CPU loads"=w430:T34[])  [unwired: 10 in]
            n208 = call "performance fg.vi"("Menu"=w428) -> ("Output"=w429:T35)  [unwired: 1 in]
            n209 = call "vision data fg.vi"("Menu"=w428) -> ()  [unwired: 1 in, 1 out]
            n210 = call "vision state fg.vi"("Menu"=w428) -> ("Enabled?"=w426:bool)  [unwired: 1 in, 1 out]
            n211 = Index Array(array=w430) -> (element=w431:T34)  [unwired: 1 in]
            n212 = Unbundle By Name(w431) -> ("Total (%)"=w423:dbl)
            n213 = Unbundle By Name(w429) -> ("Vision mSPI"=w424:u32, "Main mSPI"=w425:u32)
            n214 = Bundle By Name(cluster=T9 {"Total (%)"=0.0, "Vision mSPI"=0, "Main mSPI"=0, "Vision"={"distance"=0.0}, "Enabled?"=FALSE}, "Total (%)"=w423, "Vision mSPI"=w424, "Main mSPI"=w425, "Vision"=cluster{"distance":dbl} {"distance"=0.0}, "Enabled?"=w426) -> (w418:T9)
            n215 = Flatten To String(anything=w418, error in (no error)=w419) -> (data string=w422:string, error out=w420:errorcluster)  [unwired: 3 out]
            n216 = call <vilib>:"NT Write String.vi"("error in"=w420, "String"=w422, "Name"="dashdata") -> ("error out"=w416:errorcluster)  [unwired: 8 in]
          }
        }
      }
      "Errors" <- w234
      n217 = while {
        stop <- TRUE stop-if-true
        # "Don't unflatten strings unless you absolutly\nhave to do so"
        n218 = call <vilib>:"NT Read Boolean.vi"("Name"="use_pg_laptop") -> ("Boolean"=w237:bool)  [unwired: 9 in, 1 out]
        n219 = case shown="False" w237 {
          frame False {
            n220 = call <vilib>:"NT Read String.vi"("Name"="test_ctrls") -> ("error out"=w243:errorcluster, "String"=w242:string)  [unwired: 9 in]
            n221 = Unflatten From String(type=T7 {"Button"=FALSE, "Switch"=FALSE, "Slider"=0.0} ("Test Controls"), binary string=w242, error in (no error)=w243) -> (value=w240:T7)  [unwired: 2 in, 2 out]
            n222 = call "test input FG.vi"("Test Controls"=w240, "Menu"=fg_getset."Set") -> ()  [unwired: 1 out]
          }
          frame True {
          }
        }
      }
      n223 = case shown="True" w233 {
        frame False {
        }
        frame True {
          n224 = call <vilib>:"NT Write String.vi"("String"="blank", "Name"="code_rev") -> ()  [unwired: 9 in, 1 out]
        }
      }
    }
  }
